vi "Init.vi"(8 "error in (no error)":errorcluster, 10 "Connection String":string, 11 "Camera in":refnum<class "Camera.lvclass">) -> (0 "error out":errorcluster, 3 "Camera out":refnum<class "Camera.lvclass">)   [LabVIEW 2020, in "CameraUSB.lvlib" / "Camera.lvclass"]
doc: "Inizialize camera object\n\n<b> ConnectionString:</b> String with parameters needed to connecting to camera. The parameters are separate by ::\nThe last parameter must be the name of provider used to comunicate with camera."
uses:
  Camera.lvclass
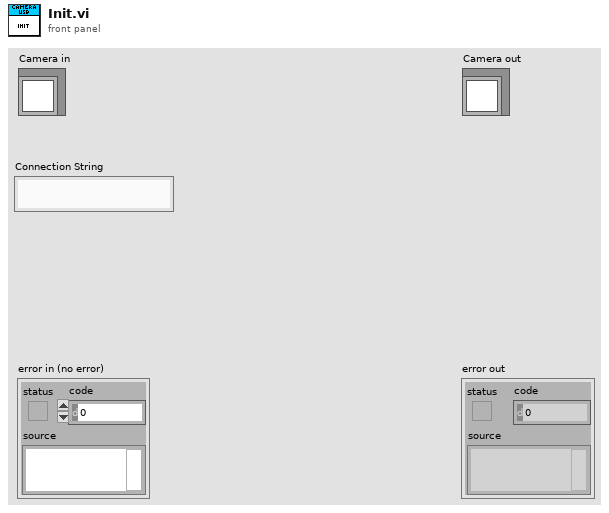
[diagram p1: front panel]
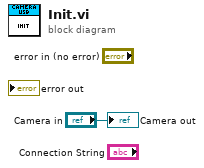
[diagram p0: block diagram]
diagram:
  "Camera out" <- "Camera in"
